vi "Getting Started.vi"() -> ()   [LabVIEW 2011]
uses:
  <vilib>/Heliosphere Research LLC/Advanced Plotting Toolkit/Advanced Plotting Toolkit.lvlib
  <vilib>/Heliosphere Research LLC/Advanced Plotting Toolkit/api_plotting/Contour_Automatic.vi
  <vilib>/Utility/sysdir.llb/System Directory Type.ctl
  <vilib>/Heliosphere Research LLC/Advanced Plotting Toolkit/properties/Line_Style.ctl
  <vilib>/Heliosphere Research LLC/Advanced Plotting Toolkit/typedefs/PlotColor.ctl
  <vilib>/Heliosphere Research LLC/Advanced Plotting Toolkit/properties/Line.ctl
  <vilib>/Heliosphere Research LLC/Advanced Plotting Toolkit/properties/Display.ctl
  <vilib>/Heliosphere Research LLC/Advanced Plotting Toolkit/api_plotting/ContourProperties.ctl
panel:
  out "Stacked Bar Plot":picture
  # "Getting Started"
  # "This VI demonstrates the basics of using the Toolkit.  It calls\nseveral plotting VIs, adjusts some parameters of the plot,\nrenders it as a LabVIEW picture and then saves it to disk.\n\nCheck out the block diagram to see how it's done."
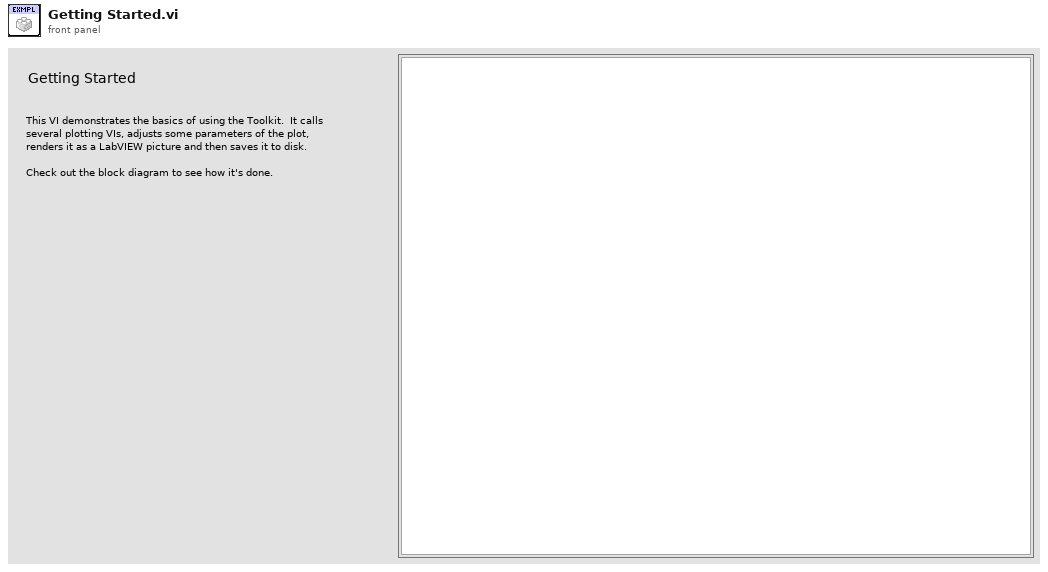
[diagram p1: front panel]
types:
  T1 = typedef "Advanced Plotting Toolkit.lvlib/ContourProperties.ctl" = cluster{"Label Contours":bool, "Line":T2, "Display":T5}
  T2 = typedef "Advanced Plotting Toolkit.lvlib/Line.ctl" = cluster{"Style":T3, "Color":T4, "Width":sgl}
  T3 = typedef "Advanced Plotting Toolkit.lvlib/Line_Style.ctl" = enum16{"Automatic", "Solid", "Dashed", "Dotted", "Dash-dot", "Invisible"}
  T4 = typedef "Advanced Plotting Toolkit.lvlib/PlotColor.ctl" = u32
  T5 = typedef "Advanced Plotting Toolkit.lvlib/Display.ctl" = cluster{"Alpha":dbl, "Z Order":dbl}
  T6 = typedef "System Directory Type.ctl" = i32
  T7 = typedef "Advanced Plotting Toolkit.lvlib/PlotID.ctl" = i32
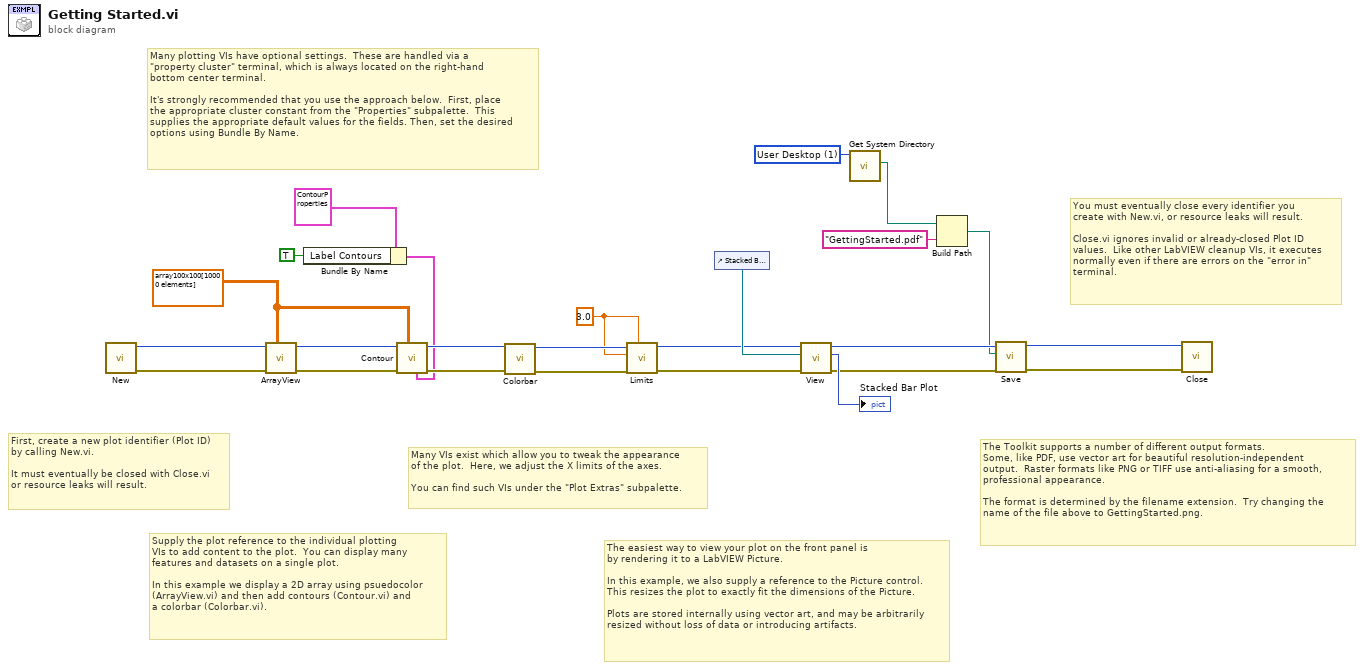
[diagram p0: block diagram]
diagram:
  w13 = T6 1 items=["User Home"=0, "User Desktop"=1, "User Documents"=2, "User Application Data"=3, "User Preferences"=4, "User Temporary"=5, "Public Documents"=6, "Public Application Data"=7, "Public Preferences"=8, "Public Cache"=13, "System Core Libraries"=9, "System Installed Libraries"=10, "Application Files"=11, "Boot Volume Root"=12] ("system directory type")
  w16 = 3.0
  w21 = sgl[][] array100x100[10000 elements] ("Array")
  # "You must eventually close every identifier you\ncreate with New.vi, or resource leaks will result.\n\nClose.vi ignores invalid or already-closed Plot ID\nvalues.  Like other LabVIEW cleanup VIs, it executes\nnormally even if there are errors on the \"error in\"\nterminal."
  # "The Toolkit supports a number of different output formats.\nSome, like PDF, use vector art for beautiful resolution-independent\noutput.  Raster formats like PNG or TIFF use anti-aliasing for a smooth,\nprofessional appearance.\n\nThe format is determined by the filename extension.  Try changing the\nname of the file above to GettingStarted.png."
  # "The easiest way to view your plot on the front panel is\nby rendering it to a LabVIEW Picture.  \n\nIn this example, we also supply a reference to the Picture control.\nThis resizes the plot to exactly fit the dimensions of the Picture.\n\nPlots are stored internally using vector art, and may be arbitrarily\nresized without loss of data or introducing artifacts."
  # "Many VIs exist which allow you to tweak the appearance\nof the plot.  Here, we adjust the X limits of the axes.\n\nYou can find such VIs under the \"Plot Extras\" subpalette."
  # "Many plotting VIs have optional settings.  These are handled via a\n\"property cluster\" terminal, which is always located on the right-hand\nbottom center terminal.\n\nIt's strongly recommended that you use the approach below.  First, place\nthe appropriate cluster constant from the \"Properties\" subpalette.  This\nsupplies the appropriate default values for the fields. Then, set the desired\noptions using Bundle By Name."
  # "Supply the plot reference to the individual plotting\nVIs to add content to the plot.  You can display many\nfeatures and datasets on a single plot.\n\nIn this example we display a 2D array using psuedocolor\n(ArrayView.vi) and then add contours (Contour.vi) and\na colorbar (Colorbar.vi)."
  # "First, create a new plot identifier (Plot ID)\nby calling New.vi.\n\nIt must eventually be closed with Close.vi\nor resource leaks will result."
  n1 = call <vilib>:"New.vi"() -> ("error out"=w18:errorcluster, "Plot ID"=w20:T7)  [unwired: 10 in]
  n2 = call <vilib>:"ArrayView.vi"("Data"=w21, "error in (no error)"=w18, "Plot ID"=w20) -> ("error out"=w17:errorcluster, "Plot ID Out"=w19:T7)  [unwired: 7 in]
  n3 = Bundle By Name(cluster=T1 {"Label Contours"=FALSE, "Line"={"Style"=enum."Automatic", "Color"=2147483647, "Width"=nan}, "Display"={"Alpha"=nan, "Z Order"=nan}} ("Contour Properties"), "Label Contours"=TRUE) -> (w2:T1)
  n4 = call-poly <vilib>:"Contour.vi"("Properties"=w2, "Z Data"=w21, "error in (no error)"=w17, "Plot ID"=w19) -> ("error out"=w3:errorcluster, "Plot ID Out"=w4:T7)  [unwired: 6 in]
  n5 = call <vilib>:"Colorbar.vi"("error in (no error)"=w3, "Plot ID"=w4) -> ("error out"=w24:errorcluster, "Plot ID Out"=w25:T7)  [unwired: 8 in]
  n6 = call <vilib>:"Limits.vi"("Y Min"=w16, "error in (no error)"=w24, "X Min"=w16, "Plot ID"=w25) -> ("error out"=w14:errorcluster, "Plot ID Out"=w15:T7)  [unwired: 6 in]
  n7 = control-ref of="Stacked Bar Plot"() -> (w22:refnum<vi>)
  n8 = call <vilib>:"View.vi"("error in (no error)"=w14, "Ref for Sizing"=w22, "Plot ID"=w15) -> ("error out"=w9:errorcluster, "Picture"=→"Stacked Bar Plot":picture, "Plot ID Out"=w10:T7)  [unwired: 6 in]
  n9 = call <vilib>:"Get System Directory.vi"("system directory type"=w13) -> ("system directory"=w12:path)  [unwired: 10 in]
  n10 = Build Path(base path=w12, name or relative path="GettingStarted.pdf") -> (appended path=w7:path)
  n11 = call <vilib>:"Save.vi"("error in (no error)"=w9, "Path"=w7, "Plot ID In"=w10) -> ("error out"=w1:errorcluster, "Plot ID Out"=w8:T7)  [unwired: 7 in]
  n12 = call <vilib>:"Close.vi"("error in (no error)"=w1, "Plot ID"=w8) -> ()  [unwired: 9 in, 1 out]
